vi "温度转换.vi"(11 "in":dbl) -> (3 "out":dbl)   [LabVIEW 2012]
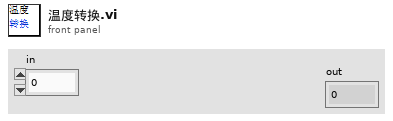
[diagram p1: front panel]
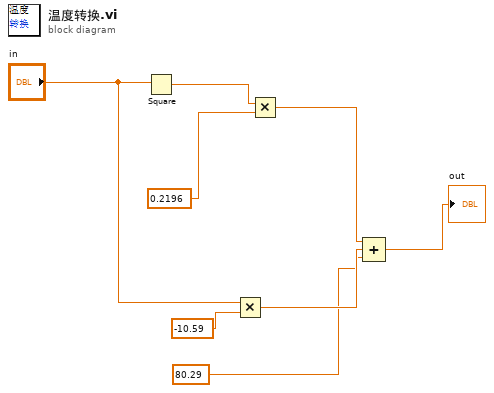
[diagram p0: block diagram]
diagram:
  n1 = Square(x="in") -> (x^2=w8:dbl)
  n2 = Multiply(x="in", y=-10.59) -> (x*y=w3:dbl)
  n3 = Multiply(x=w8, y=0.2196) -> (x*y=w4:dbl)
  n4 = Compound Arithmetic op=ADD(w4, w3, 80.29) -> (→"out":dbl)
